vi "MT Generate ASK system parameters (map).vi"(0 "samples per symbol (16)":i32=16, 5 "symbol values":i32[](array[numeric]), 11 "error in (no error)":errorcluster) -> (6 "ASK system parameters":T1 {"symbol map" format="%.3f"}, 8 "bits per symbol":i32, 15 "error out":errorcluster)   [LabVIEW 2020, in "niDMT.lvlib"]
doc: "This polymorphic instance calculates parameters for use with either the MT Modulate ASK VI or the MT Demodulate ASK VI. It accepts an array of <B>symbol values</B> that explicitly specifies the symbol positions of a symbol map with symbols that are evenly distributed between 0 and 1."
uses:
  <vilib>/addons/Modulation/niDMT.lvlib
  <vilib>/addons/Modulation/Digital/Support/Controls/ASK system parameters.ctl
  <vilib>/addons/Modulation/niAMT.lvlib
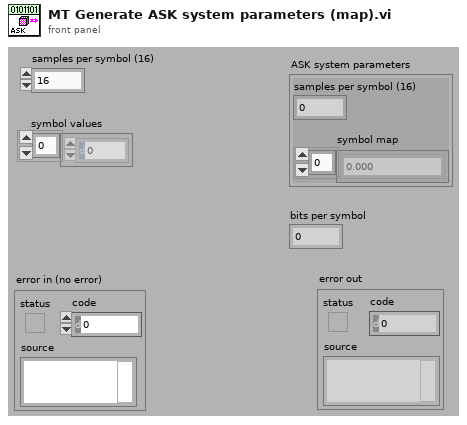
[diagram p1: front panel]
types:
  T1 = cluster{"samples per symbol (16)":i32, "symbol map":cdb[]}
  T2 = typedef "niDMT.lvlib/ASK system parameters.ctl" = cluster{"samples per symbol (16)":i32, "symbol map":cdb[]}
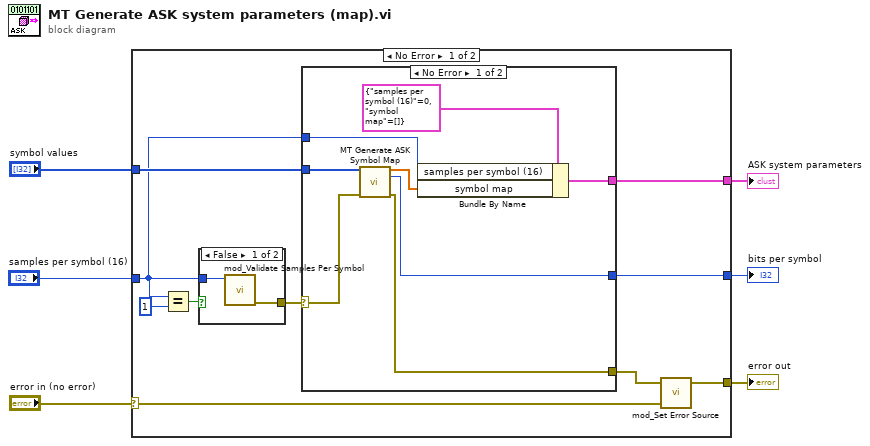
[diagram p0: block diagram]
diagram:
  n1 = case shown="No Error" "error in (no error)" {
    selector: "error in (no error)" -> [w12 w28]
    tunnel: [w16 _] -> w6
    tunnel: [w15 _] -> w5
    tunnel: [w11 w28] -> w4
    tunnel: "symbol values" -> [w14 _]
    tunnel: "samples per symbol (16)" -> [w9 _]
    frame No Error {
      n2 = Equal?(x=w9, y=1) -> (x = y?=w7:bool)
      n3 = case shown="False" w7 {
        tunnel: w9 -> [w18 _]
        tunnel: [w17 _] -> w13
        frame False {
          n4 = call <vilib>:"mod_Validate Samples Per Symbol.vi"("Samples Per Symbol"=w18) -> ("error out"=w17:errorcluster)  [unwired: 10 out]
        }
        frame True {
        }
      }
      n5 = case shown="No Error" w13 {
        selector: w13 -> [w20 w27]
        tunnel: [w25 _] -> w16
        tunnel: [w24 _] -> w15
        tunnel: [w23 w27] -> w10
        tunnel: w14 -> [w22 _]
        tunnel: w9 -> [w21 _]
        frame No Error {
          n6 = call <vilib>:"MT Generate ASK Symbol Map.vi"("symbol values"=w22, "error in (no error)"=w20) -> ("symbol map"=w26:cdb[], "bits per symbol"=w24:i32, "error out"=w23:errorcluster)  [unwired: 11 out]
          n7 = Bundle By Name(cluster=T2 {"samples per symbol (16)"=0, "symbol map"=[]} ("ASK System Parameters"), "samples per symbol (16)"=w21, "symbol map"=w26) -> (w25:T2)
        }
        frame Error {
        }
      }
      n8 = call <vilib>:"mod_Set Error Source.vi"("initial error in (no error)"=w12, "final error in (no error)"=w10) -> ("error out"=w11:errorcluster)  [unwired: 3 out]
    }
    frame Error {
    }
  }
  "ASK system parameters" <- w6
  "bits per symbol" <- w5
  "error out" <- w4
